vi "clFile_contentLen.vi"(11 "clFile.lvclass":refnum<class "clFile.lvclass">) -> (3 "length":u32)   [LabVIEW 2021, in "vi_lib.lvlib" / "clFile.lvclass"]
uses:
  clFile.lvclass
  clFile.lvclass/clFile.ctl
panel:
  out "clFile.lvclass":refnum<class "clFile.lvclass">
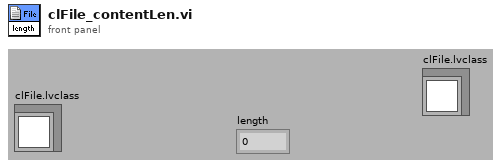
[diagram p1: front panel]
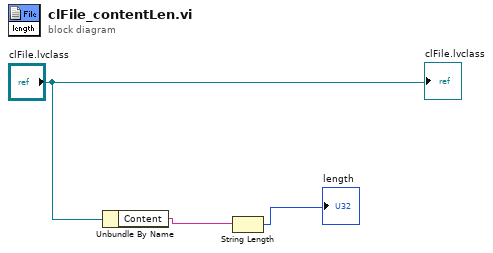
[diagram p0: block diagram]
diagram:
  n1 = Unbundle By Name("clFile.lvclass") -> ("Content"=w1:string)
  n2 = String Length(string=w1) -> (length=→"length":i32)
  "clFile.lvclass" <- "clFile.lvclass"
